vi "2_AdvancedDemo_HHHisto.vi"() -> ()   [LabVIEW 2020]
uses:
  Types/HH_InputChannel.ctl
  Types/HH_UIThread_Cmds.ctl
  Types/HH_UIThread_Data.ctl
  _lib/PQ/HydraHarp/HH_InitInfo.ctl
  _lib/PQ/HydraHarp/HH_RefSource.ctl
  _lib/PQ/HydraHarp/HH_MeasMode.ctl
  <vilib>/Utility/error.llb/DialogType.ctl
  _lib/PQ/HydraHarp/hhlib_x86_x64_UIThread.llb/HH_DllPath_global.vi
  <vilib>/Utility/error.llb/Error Cluster From Error Code.vi
  _lib/PQ/HydraHarp/HH_LibVersion_global.vi
  <vilib>/ErrorRing/Error Ring.xnode
panel:
  in  "Settings":bool=TRUE
  in  "Run continuously":bool=TRUE caption="Conti."
  in  "Start":bool
  in  "Scale":bool
  out "CountRates":i32[](graph)
  in  "HistoLength":i32(ring)=6 caption="Num Bins" items=["1024", "2048", "4096", "8192", "16384", "32768", "65536"]
  in  "OvlLevel":u32=4294967295 caption="Ovl.Level" min=1 step=1
  in  "StopOvl.":bool=TRUE
  in  "AcqTime":i32=1000 caption="Acqu.     ms" min=1 max=360000000 step=1
  in  "Binning":i32(ring) caption="Resol.      ps" items=["1", "2", "4", "8", "16", "32", "64", "128", "256", "512", "1024", "2048", "4096", "8192", "16384", "32768", "65536", "131072", "262144", "524288", "1048576", "2097152", "4194304", "8388608", "16777216", "33554432"]
  in  "HistoOffset":i32 caption="Offset      ns" min=0 max=500000 step=1
  out "HistoGraph":T1(graph)={0.0, "Resolution"=0.001, "Histogram"=array8x1024[8192 elements]}
  in  "SyncZeroX":i32=10 caption="ZeroCr.  mV" min=0 max=40 step=1
  in  "SyncDivider":i32(ring)=3 caption="Divider" items=["1", "2", "4", "8", "16"]
  in  "SyncOffset":i32 caption="Offset      ps" min=-99999 max=99999 step=1
  in  "SyncLevel":i32=50 caption="Level      mV" min=0 max=1000 step=1
  in  "Channels":T2[](array[typedef])=[{"Name"="Inp.Chan 1", "Enable"=TRUE, "Offset"=0, "CFDLevel"=50, "ZeroX"=10}, {"Name"="Inp.Chan 2", "Enable"=TRUE, "Offset"=0, "CFDLevel"=50, "ZeroX"=10}, {"Name"="Inp.Chan 3", "Enable"=TRUE, "Offset"=0, "CFDLevel"=50, "ZeroX"=10}, {"Name"="Inp.Chan 4", "Enable"=TRUE, "Offset"=0, "CFDLevel"=50, "ZeroX"=10}, {"Name"="Inp.Chan 5", "Enable"=TRUE, "Offset"=0, "CFDLevel"=50, "ZeroX"=10}, {"Name"="Inp.Chan 6", "Enable"=TRUE, "Offset"=0, "CFDLevel"=50, "ZeroX"=10}, {"Name"="Inp.Chan 7", "Enable"=TRUE, "Offset"=0, "CFDLevel"=50, "ZeroX"=10}, {"Name"="Inp.Chan 8", "Enable"=TRUE, "Offset"=0, "CFDLevel"=50, "ZeroX"=10}] {"ZeroX" min=0 max=40 step=1; "Offset" min=-99999 max=99999 step=1; "CFDLevel" min=0 max=1000 step=1}
  out "SyncRate":string="Sync Rate: 0 cps\n"
  out "OverFlow":bool caption="Overflow:"
  out "Status":string="Initialized!"
  # "Histogram"
  # "Sync"
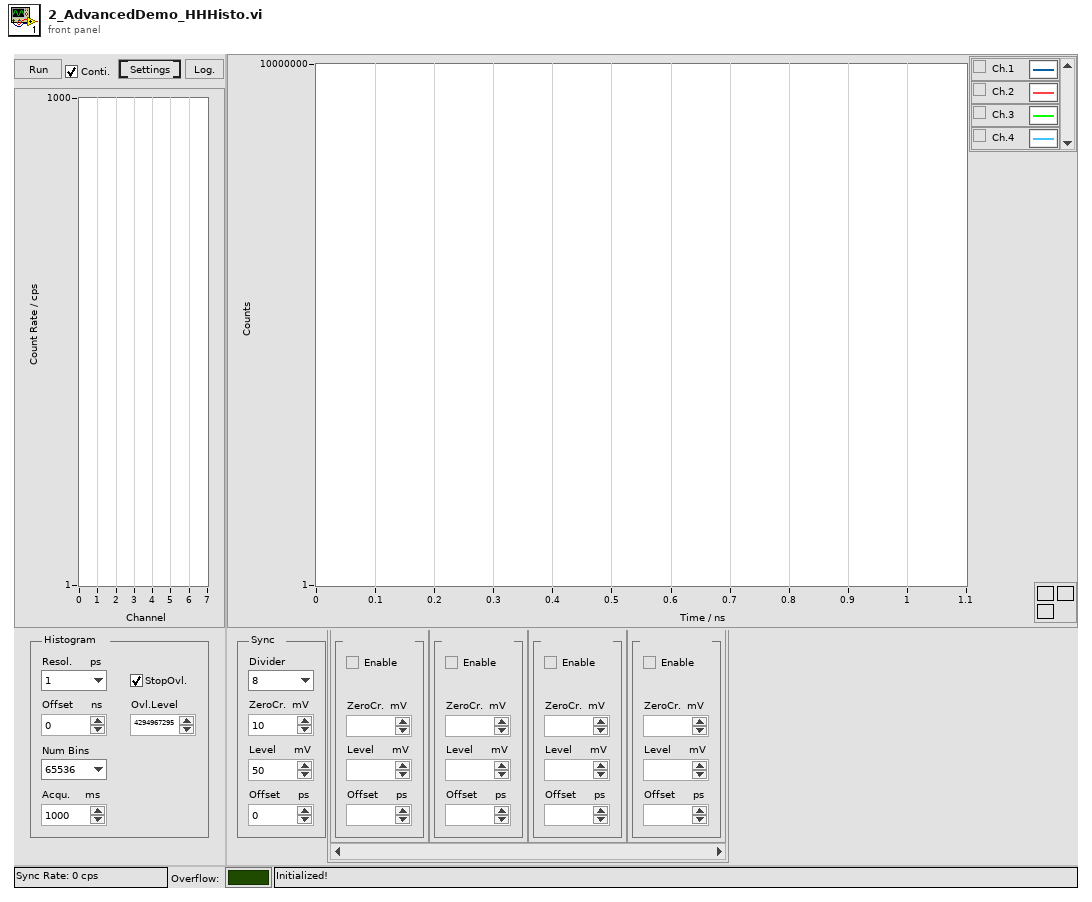
[diagram p1: front panel]
types:
  T1 = cluster{dbl, "Resolution":dbl, "Histogram":u32[][]}
  T2 = typedef "HH_InputChannel.ctl" = cluster{"Name":string, "Enable":bool, "Offset":i32, "CFDLevel":i32, "ZeroX":i32}
  T3 = typedef "HH_UIThread_Data.ctl" = cluster{"Init Info":T4, "DevIdx":i32, "SyncDivider":i32, "SyncOffset":i32, "SyncLevel":i32, "Channels":T2[], "CurrentChannels":i32[], "AcqTime":i32, "Binning":i32, "HistoOffset":i32, "HistoLen":i32, "StopOvl.":bool, "OvlLevel":u32, "StartMeas":bool, "HistoLength":i32, "Resolution":dbl, "Run cont.":bool, "Status":string, "SyncRate":i32, "BitShift":i32, "HistoAcqTime":dbl, "SyncZeroX":i32, "SyncRateStart":i32}
  T4 = typedef "HH_InitInfo.ctl" = cluster{"Library Version":string, "Serial No.":string, "Model":string, "Partnum":string, "Version":string, "features":i32, "nchannels":i32, "nummod":i32, "Model Codes":i32[], "Version Codes":i32[], "Base Resolution":dbl, "Bin Steps":i32}
  T5 = typedef "HH_UIThread_Cmds.ctl" = enum16{"Idle", "Init", "SetInpChanEnable", "SetInpChanOffset", "SetInpChanTrg", "SetSyncDivider", "SetSyncTrg", "SetSyncOffset", "SetBinning", "SetHistoOffset", "SetHistoLen", "SetStopOvl", "SetBitShift", "SetHistoAcqTime", "GetRates", "StartMeas", "StopMeas", "AbortMeas", "GetResolution", "GetHisto", "ReadFiFo", "WriteStatus", "Resize", "EnableControls", "DisableControls", "Error", "Exit"}
  T6 = enum8{"Enabled", "Disabled", "Disabled and Grayed Out"}
  T7 = typedef "HH_MeasMode.ctl" = i32
  T8 = typedef "HH_RefSource.ctl" = enum16{"internal", "external"}
  T9 = typedef "DialogType.ctl" = u16
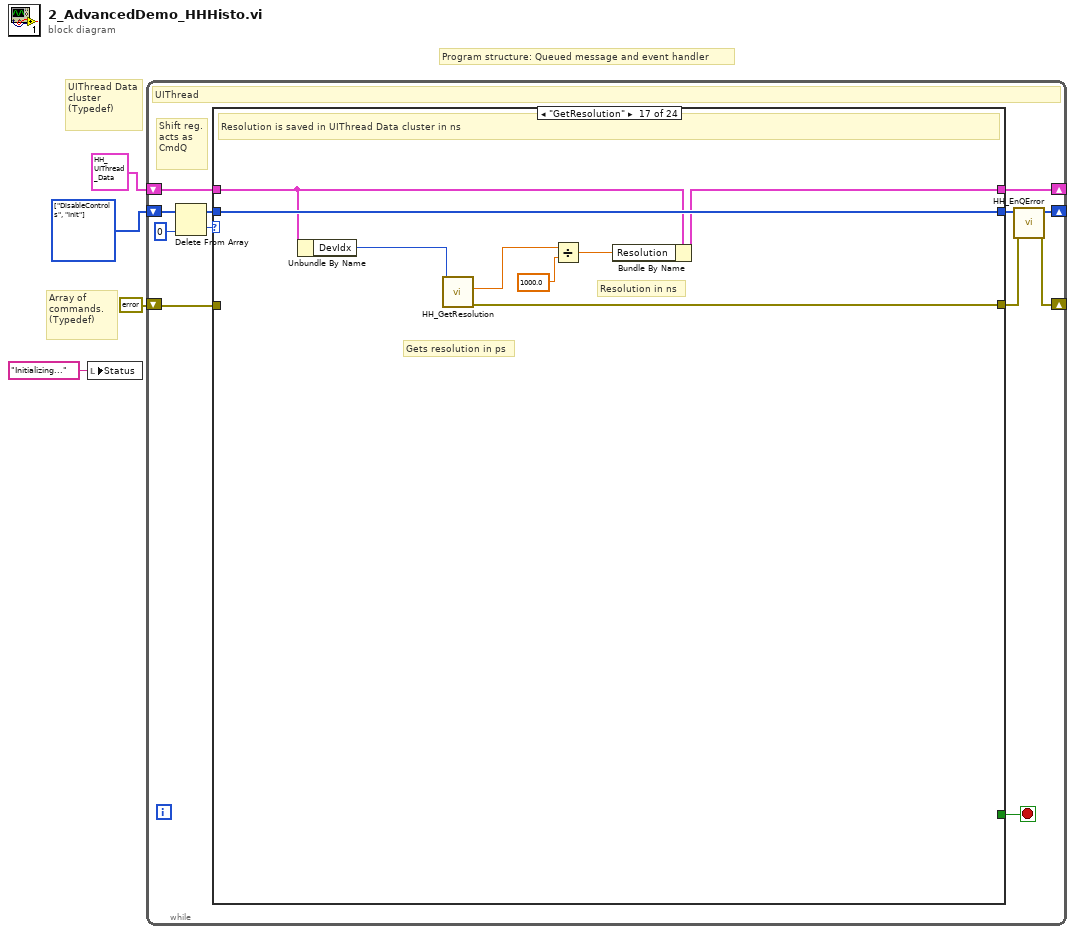
[diagram p0: block diagram]
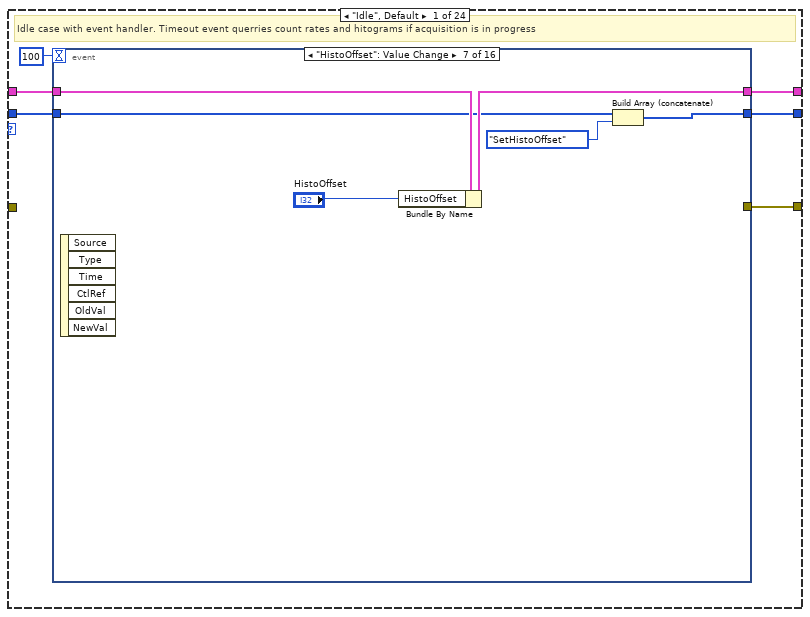
[diagram p2: hidden frame]
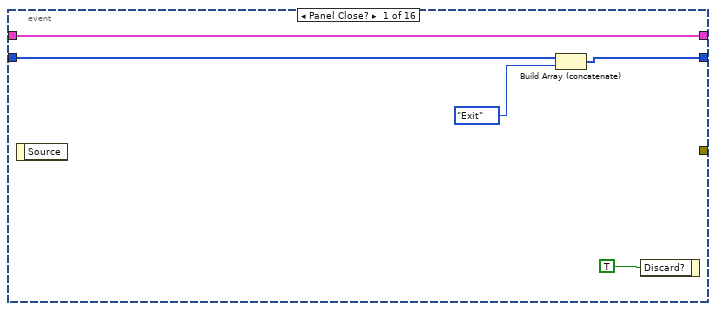
[diagram p3: hidden frame]
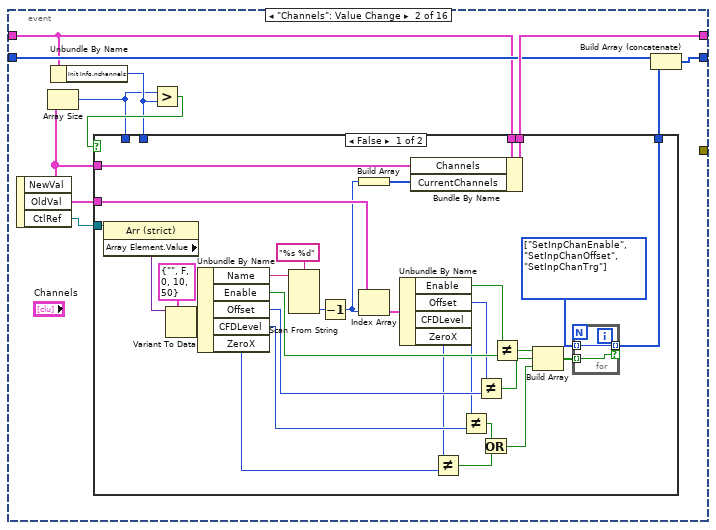
[diagram p4: hidden frame]
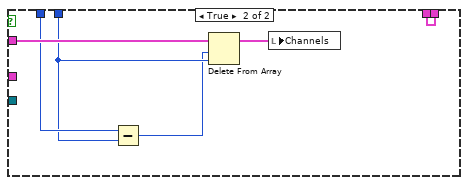
[diagram p5: hidden frame]
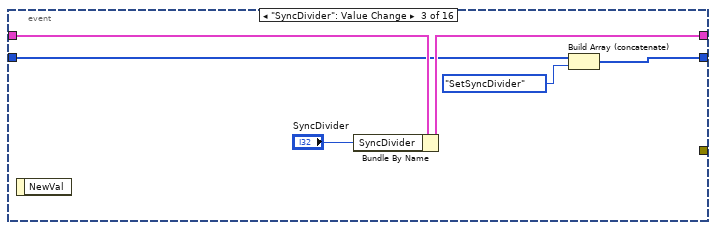
[diagram p6: hidden frame]
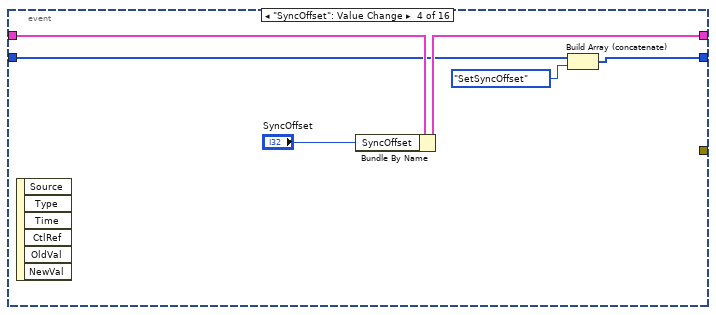
[diagram p7: hidden frame]
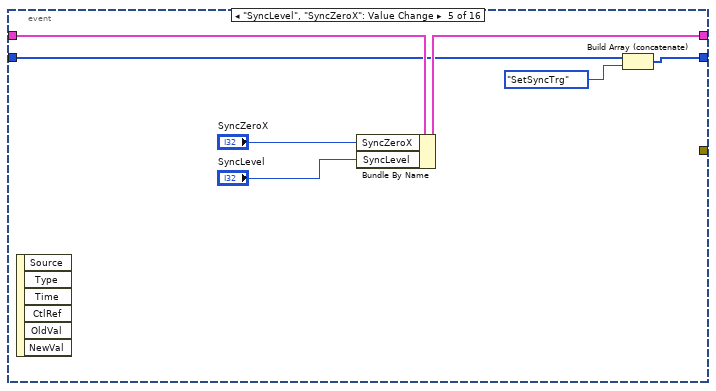
[diagram p8: hidden frame]
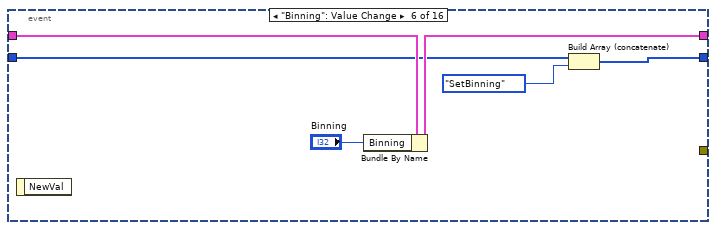
[diagram p9: hidden frame]
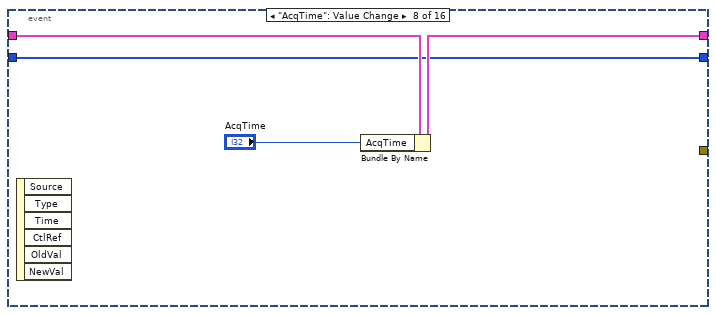
[diagram p10: hidden frame]
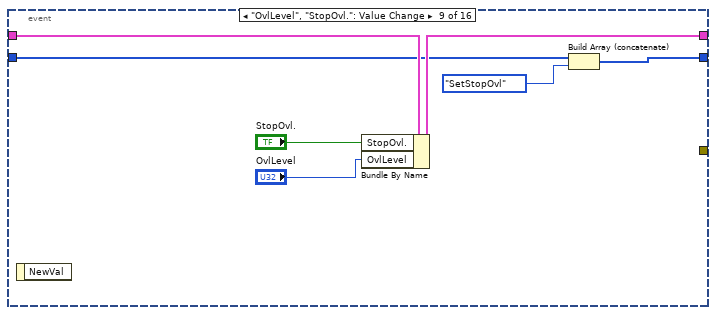
[diagram p11: hidden frame]
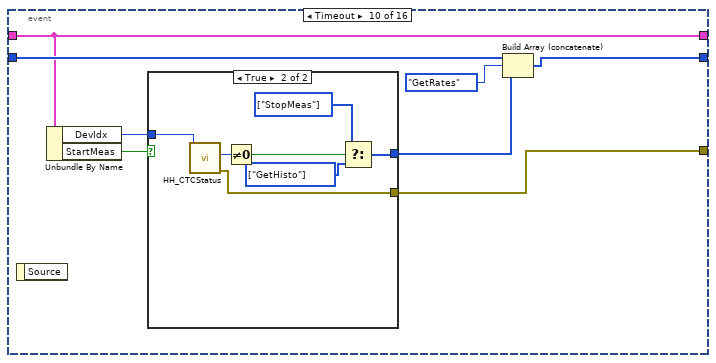
[diagram p12: hidden frame]
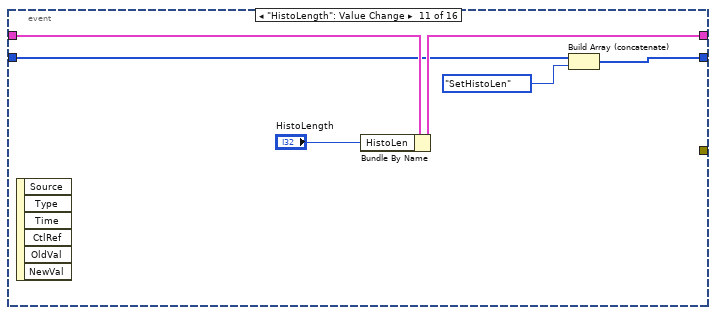
[diagram p14: hidden frame]
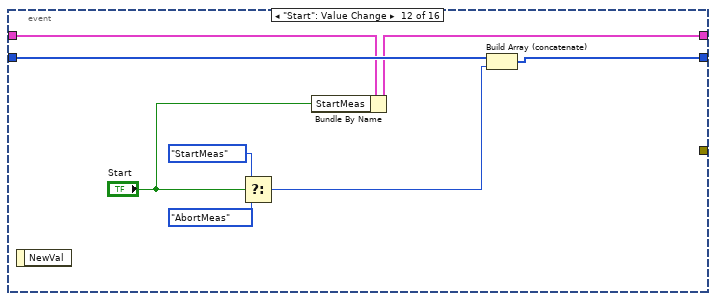
[diagram p15: hidden frame]
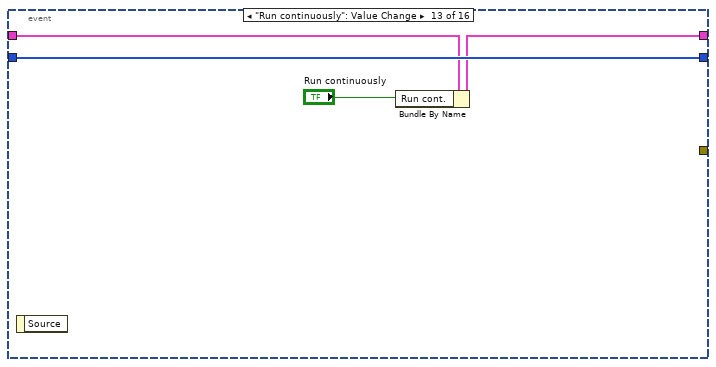
[diagram p16: hidden frame]
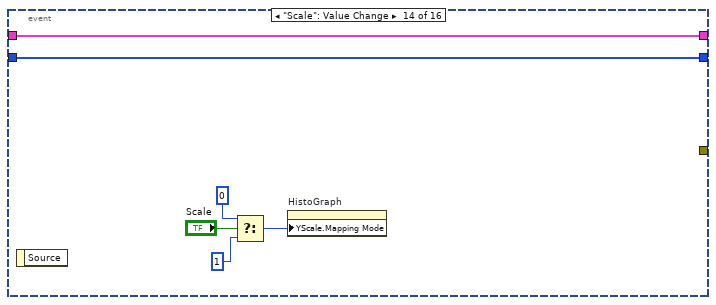
[diagram p17: hidden frame]
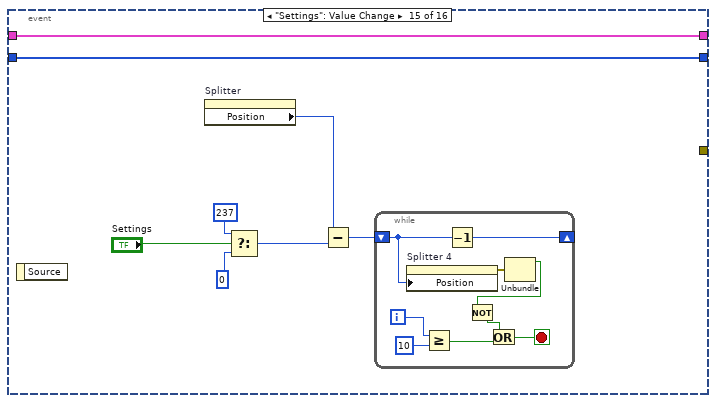
[diagram p18: hidden frame]
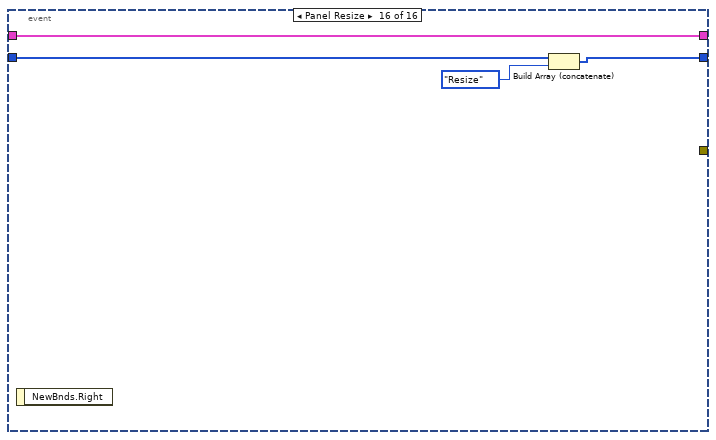
[diagram p19: hidden frame]
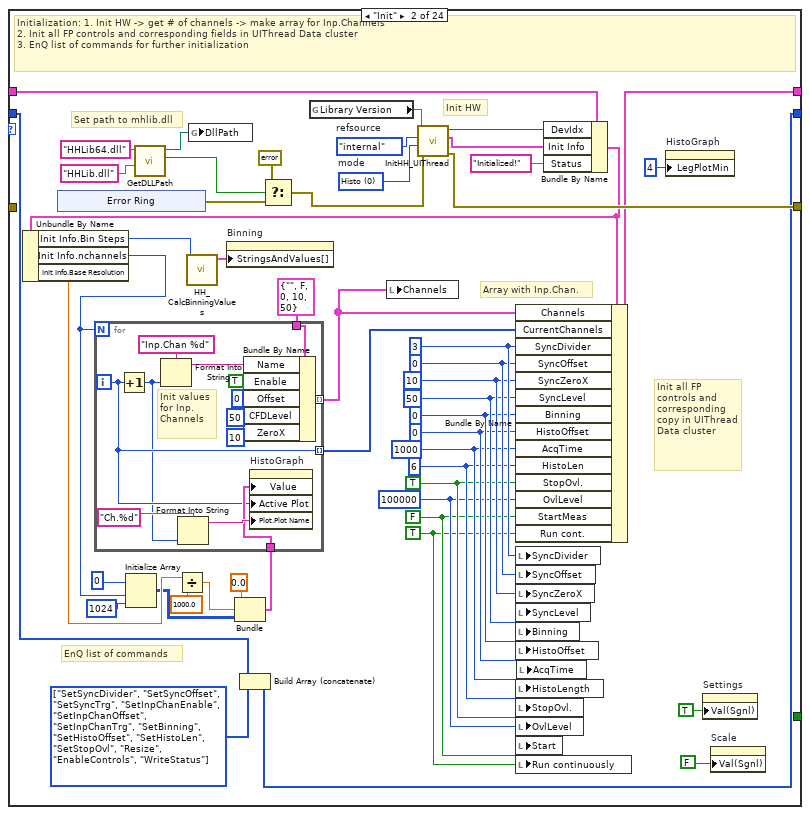
[diagram p20: hidden frame]
diagram:
  w3 = T5[] [enum."DisableControls", enum."Init"] items=["Idle", "Init", "SetInpChanEnable", "SetInpChanOffset", "SetInpChanTrg", "SetSyncDivider", "SetSyncTrg", "SetSyncOffset", "SetBinning", "SetHistoOffset", "SetHistoLen", "SetStopOvl", "SetBitShift", "SetHistoAcqTime", "GetRates", "StartMeas", "StopMeas", "AbortMeas", "GetResolution", "GetHisto", "ReadFiFo", "WriteStatus", "Resize", "EnableControls", "DisableControls", "Error", "Exit"]
  # "Array of commands.\n(Typedef)"
  # "Program structure: Queued message and event handler"
  # "UIThread Data cluster\n(Typedef)"
  n1 = local write "Status"("Initializing..." ("Status")) -> ()
  n2 = while {
    shift-right: [w5] -> _
    shift-left: w3 -> [w12]
    shift-right: [w15] -> _
    shift-left: T3 {"Init Info"={"Library Version"="", "Serial No."="", "Model"="", "Partnum"="", "Version"="", "features"=0, "nchannels"=0, "nummod"=0, "Model Codes"=[], "Version Codes"=[], "Base Resolution"=0.0, "Bin Steps"=0}, "DevIdx"=0, "SyncDivider"=1, "SyncOffset"=0, "SyncLevel"=50, "Channels"=[], "CurrentChannels"=[], "AcqTime"=1, "Binning"=1, "HistoOffset"=1, "HistoLen"=1024, "StopOvl."=FALSE, "OvlLevel"=1024, "StartMeas"=FALSE, "HistoLength"=0, "Resolution"=0.0, "Run cont."=FALSE, "Status"="", "SyncRate"=0, "BitShift"=0, "HistoAcqTime"=0.0, "SyncZeroX"=10, "SyncRateStart"=0} -> [w14]
    shift-right: [w7] -> _
    shift-left: errorcluster {"status"=FALSE, "code"=0, "source"=""} ("error IO") -> [w13]
    stop <- w16 stop-if-true
    # "Shift reg.\nacts as\nCmdQ"
    # "UIThread"
    n3 = Delete From Array(array=w12, index=0) -> (deleted portion=w10:T5, array with subset deleted=w9:T5[])  [unwired: 1 in]
    n4 = case shown="\"GetResolution\"" w10 {
      tunnel: [w22 w221 w249 w263 w277 w294 w303 w305 w312 w320 w328 w333 w345 w360 w368 w382 w396 w421 w446 w459 w466 w478 w484 w488] -> w6
      tunnel: [_ _ _ _ _ _ _ _ _ _ _ _ _ _ _ _ _ _ _ _ _ _ _ TRUE] -> w16
      tunnel: [w21 w201 w252 w266 w280 w296 w304 w309 w316 w321 w323 w334 w344 w366 w371 w385 w392 w420 w445 w447 w465 w477 w485 w491] -> w15
      tunnel: w14 -> [w20 w206 w252 w266 w280 w296 w304 w309 w316 w321 w324 w334 w344 w366 w372 w386 w393 w420 w445 w447 w465 w477 w485 w491]
      tunnel: [w17 w224 w250 w264 w278 w292 w302 w308 w315 w319 w327 w332 w343 w365 w374 w388 w394 w416 _ _ _ _ _ w489] -> w8
      tunnel: w13 -> [_ _ _ _ _ _ _ _ _ _ _ _ _ _ _ _ _ _ _ _ _ _ w486 _]
      tunnel: w9 -> [w19 w223 w249 w263 w277 w294 w303 w305 w311 w320 w328 w333 w345 w361 w369 w383 w396 w421 w446 w459 w466 w478 _ w488]
      frame "Idle", Default {
        # "Idle case with event handler. Timeout event querries count rates and hitograms if acquisition is in progress"
        n5 = event shown="[6] \"HistoOffset\": Value Change" {
          selector: _ -> [_ _ _ _ _ _ _ _ _ _ _ _ _ _ _ _]
          dyn-events: _ -> [_ _ _ _ _ _ _ _ _ _ _ _ _ _ _ _]
          timeout: 100 -> [_ _ _ _ _ _ _ _ _ _ _ _ _ _ _ _]
          tunnel: [w23 w33 w77 w83 w90 w97 w103 w108 w114 w124 w135 w143 w151 w157 w165 w175] -> w22
          tunnel: [w26 w36 w81 w87 w94 w100 w106 w110 w117 w123 w138 w141 w149 w156 w164 w178] -> w21
          tunnel: w20 -> [w26 w32 w82 w88 w95 w101 w107 w111 w118 w123 w139 w142 w150 w156 w164 w178]
          tunnel: w19 -> [w25 w35 w79 w85 w92 w99 w105 w108 w116 w126 w137 w145 w151 w157 w165 w176]
          tunnel: [_ _ _ _ _ _ _ _ _ w119 _ _ _ _ _ _] -> w17
          event Panel Close? {
            n6 = event-data() -> ()  [unwired: 1 in, 1 out]
            n7 = Build Array (concatenate)(w25, HH_UIThread_Cmds."Exit") -> (w23:T5[])
            n8 = event-data("Discard?"=TRUE) -> ()  [unwired: 1 in, 1 out]
          }
          event "Channels": Value Change {
            n9 = event-data() -> ("NewVal"=w31:T2[], "OldVal"=w37:T2[], "CtlRef"=w38:refnum<vi>)  [unwired: 1 in]
            n10 = Array Size(array=w31) -> (size(s)=w28:i32)
            n11 = Unbundle By Name(w32) -> ("Init Info.nchannels"=w29:i32)
            n12 = Greater?(x=w28, y=w29) -> (0:w30:bool)
            n13 = case shown="False" w30 {
              tunnel: w38 -> [w68 _]
              tunnel: w37 -> [w62 _]
              tunnel: [w45 w76] -> w36
              tunnel: [w43 _] -> w34
              tunnel: w32 -> [w40 w76]
              tunnel: w31 -> [w39 w75]
              tunnel: w29 -> [_ w73]
              tunnel: w28 -> [_ w74]
              frame False {
                w46 = T5[] [enum."SetInpChanEnable", enum."SetInpChanOffset", enum."SetInpChanTrg"] items=["Idle", "Init", "SetInpChanEnable", "SetInpChanOffset", "SetInpChanTrg", "SetSyncDivider", "SetSyncTrg", "SetSyncOffset", "SetBinning", "SetHistoOffset", "SetHistoLen", "SetStopOvl", "SetBitShift", "SetHistoAcqTime", "GetRates", "StartMeas", "StopMeas", "AbortMeas", "GetResolution", "GetHisto", "ReadFiFo", "WriteStatus", "Resize", "EnableControls", "DisableControls", "Error", "Exit"]
                n14 = property class="Arr (strict)"(reference=w68) -> ("Array Element.Value"=w67:variant)  [unwired: 1 in, 2 out]
                n15 = Variant To Data(type=T2 {"Name"="", "Enable"=FALSE, "Offset"=0, "CFDLevel"=10, "ZeroX"=50} ("Channel"), Variant=w67) -> (data=w44:T2)  [unwired: 1 in, 1 out]
                n16 = Unbundle By Name(w44) -> ("Name"=w65:string, "Enable"=w59:bool, "Offset"=w57:i32, "CFDLevel"=w55:i32, "ZeroX"=w53:i32)
                n17 = Scan From String(format string="%s %d", input string=w65) -> (output 2=w63:i32)  [unwired: 5 in, 3 out]
                n18 = Decrement(x=w63) -> (x-1=w42:i32)
                n19 = Build Array(w42) -> (w41:i32[])
                n20 = Index Array(array=w62, index=w42) -> (element=w61:T2)
                n21 = Unbundle By Name(w61) -> ("Enable"=w60:bool, "Offset"=w58:i32, "CFDLevel"=w56:i32, "ZeroX"=w54:i32)
                n22 = Bundle By Name(cluster=w40, "Channels"=w39, "CurrentChannels"=w41) -> (w45:T3)
                n23 = Not Equal?(x=w54, y=w53) -> (x != y?=w48:bool)
                n24 = Not Equal?(x=w56, y=w55) -> (x != y?=w49:bool)
                n25 = Not Equal?(x=w58, y=w57) -> (x != y?=w51:bool)
                n26 = Or(x=w49, y=w48) -> (x .or. y?=w47:bool)
                n27 = Not Equal?(x=w60, y=w59) -> (x != y?=w52:bool)
                n28 = Build Array(w52, w51, w47) -> (w50:bool[])
                n29 = for {
                  tunnel: w50 -> [w69] mode=indexing
                  tunnel: w46 -> [w70] mode=indexing
                  tunnel: [w70] -> w43 mode=indexing if=w69
                }
              }
              frame True {
                n30 = Subtract(x=w74, y=w73) -> (x-y=w72:i32)
                n31 = Delete From Array(array=w75, length=w72, index=w73) -> (array with subset deleted=w71:T2[])  [unwired: 1 out]
                n32 = local write "Channels"(w71) -> ()
              }
            }
            n33 = Build Array (concatenate)(w35, w34) -> (w33:T5[])
          }
          event "SyncDivider": Value Change {
            n34 = event-data() -> ()  [unwired: 1 in, 1 out]
            n35 = Bundle By Name(cluster=w82, "SyncDivider"="SyncDivider") -> (w81:T3)
            n36 = Build Array (concatenate)(w79, HH_UIThread_Cmds."SetSyncDivider") -> (w77:T5[])
          }
          event "SyncOffset": Value Change {
            n37 = event-data() -> ()  [unwired: 1 in, 6 out]
            n38 = Bundle By Name(cluster=w88, "SyncOffset"="SyncOffset") -> (w87:T3)
            n39 = Build Array (concatenate)(w85, HH_UIThread_Cmds."SetSyncOffset") -> (w83:T5[])
          }
          event "SyncLevel", "SyncZeroX": Value Change {
            n40 = event-data() -> ()  [unwired: 1 in, 6 out]
            n41 = Bundle By Name(cluster=w95, "SyncZeroX"="SyncZeroX", "SyncLevel"="SyncLevel") -> (w94:T3)
            n42 = Build Array (concatenate)(w92, HH_UIThread_Cmds."SetSyncTrg") -> (w90:T5[])
          }
          event "Binning": Value Change {
            n43 = event-data() -> ()  [unwired: 1 in, 1 out]
            n44 = Bundle By Name(cluster=w101, "Binning"="Binning") -> (w100:T3)
            n45 = Build Array (concatenate)(w99, HH_UIThread_Cmds."SetBinning") -> (w97:T5[])
          }
          event "HistoOffset": Value Change {
            n46 = event-data() -> ()  [unwired: 1 in, 6 out]
            n47 = Bundle By Name(cluster=w107, "HistoOffset"="HistoOffset") -> (w106:T3)
            n48 = Build Array (concatenate)(w105, HH_UIThread_Cmds."SetHistoOffset") -> (w103:T5[])
          }
          event "AcqTime": Value Change {
            n49 = event-data() -> ()  [unwired: 1 in, 6 out]
            n50 = Bundle By Name(cluster=w111, "AcqTime"="AcqTime") -> (w110:T3)
          }
          event "OvlLevel", "StopOvl.": Value Change {
            n51 = event-data() -> ()  [unwired: 1 in, 1 out]
            n52 = Bundle By Name(cluster=w118, "StopOvl."="StopOvl.", "OvlLevel"="OvlLevel") -> (w117:T3)
            n53 = Build Array (concatenate)(w116, HH_UIThread_Cmds."SetStopOvl") -> (w114:T5[])
          }
          event Timeout {
            n54 = event-data() -> ()  [unwired: 1 in, 1 out]
            n55 = Unbundle By Name(w123) -> ("DevIdx"=w121:i32, "StartMeas"=w122:bool)
            n56 = case shown="True" w122 {
              tunnel: w121 -> [_ w133]
              tunnel: [_ w131] -> w120
              tunnel: [_ w128] -> w119
              frame False {
              }
              frame True {
                w129 = T5[] [enum."GetHisto"] items=["Idle", "Init", "SetInpChanEnable", "SetInpChanOffset", "SetInpChanTrg", "SetSyncDivider", "SetSyncTrg", "SetSyncOffset", "SetBinning", "SetHistoOffset", "SetHistoLen", "SetStopOvl", "SetBitShift", "SetHistoAcqTime", "GetRates", "StartMeas", "StopMeas", "AbortMeas", "GetResolution", "GetHisto", "ReadFiFo", "WriteStatus", "Resize", "EnableControls", "DisableControls", "Error", "Exit"]
                w130 = T5[] [enum."StopMeas"] items=["Idle", "Init", "SetInpChanEnable", "SetInpChanOffset", "SetInpChanTrg", "SetSyncDivider", "SetSyncTrg", "SetSyncOffset", "SetBinning", "SetHistoOffset", "SetHistoLen", "SetStopOvl", "SetBitShift", "SetHistoAcqTime", "GetRates", "StartMeas", "StopMeas", "AbortMeas", "GetResolution", "GetHisto", "ReadFiFo", "WriteStatus", "Resize", "EnableControls", "DisableControls", "Error", "Exit"]
                n57 = call "HH_CTCStatus.vi"("devidx"=w133) -> ("error out"=w128:errorcluster, "ctcstatus"=w132:i32)  [unwired: 8 in, 1 out]
                n58 = Not Equal To 0?(x=w132) -> (x != 0?=w127:bool)
                n59 = Select(t=w130, s=w127, f=w129) -> (s? t:f=w131:T5[])
              }
            }
            n60 = Build Array (concatenate)(w126, HH_UIThread_Cmds."GetRates", w120) -> (w124:T5[])
          }
          event "HistoLength": Value Change {
            n61 = event-data() -> ()  [unwired: 1 in, 6 out]
            n62 = Bundle By Name(cluster=w139, "HistoLen"="HistoLength") -> (w138:T3)
            n63 = Build Array (concatenate)(w137, HH_UIThread_Cmds."SetHistoLen") -> (w135:T5[])
          }
          event "Start": Value Change {
            n64 = event-data() -> ()  [unwired: 1 in, 1 out]
            n65 = Select(t=HH_UIThread_Cmds."StartMeas", s="Start", f=HH_UIThread_Cmds."AbortMeas") -> (s? t:f=w144:T5)
            n66 = Bundle By Name(cluster=w142, "StartMeas"="Start") -> (w141:T3)
            n67 = Build Array (concatenate)(w145, w144) -> (w143:T5[])
          }
          event "Run continuously": Value Change {
            n68 = event-data() -> ()  [unwired: 1 in, 1 out]
            n69 = Bundle By Name(cluster=w150, "Run cont."="Run continuously") -> (w149:T3)
          }
          event "Scale": Value Change {
            n70 = event-data() -> ()  [unwired: 1 in, 1 out]
            n71 = Select(t=u8 0 ("Y Scale.Mapping Mode"), s="Scale", f=u8 1 ("Y Scale.Mapping Mode")) -> (s? t:f=w152:u8)
            n72 = property on="HistoGraph" class="WFGraph (strict)"("YScale.Mapping Mode"=w152) -> ()  [unwired: 2 in, 2 out]
          }
          event "Settings": Value Change {
            n73 = event-data() -> ()  [unwired: 1 in, 1 out]
            n74 = property on="Splitter" class="Splitter"() -> ("Position"=w163:i32)  [unwired: 2 in, 2 out]
            n75 = Select(t=237 ("PosT"), s="Settings", f=0 ("PosF")) -> (s? t:f=w160:i32)
            n76 = Subtract(x=w163, y=w160) -> (x-y=w159:i32)
            n77 = while {
              shift-right: [w174] -> _
              shift-left: w159 -> [w167]
              i -> [w173]
              stop <- w170 stop-if-true
              n78 = property on="Splitter 4" class="Splitter"("Position"=w167) -> (error out=w166:errorcluster)  [unwired: 2 in, 1 out]
              n79 = Greater Or Equal?(x=w173, y=10) -> (x >= y?=w171:bool)
              n80 = Decrement(x=w167) -> (x-1=w174:i32)
              n81 = Unbundle(w166) -> ("status"=w169:bool)  [unwired: 2 out]
              n82 = Not(x=w169) -> (.not. x?=w168:bool)
              n83 = Or(x=w168, y=w171) -> (x .or. y?=w170:bool)
            }
          }
          event Panel Resize {
            n84 = event-data() -> ()  [unwired: 1 in, 1 out]
            n85 = Build Array (concatenate)(w176, HH_UIThread_Cmds."Resize") -> (w175:T5[])
          }
        }
      }
      frame "Init" {
        w193 = T7 0 items=["Histo"=0, "T2"=2, "T3"=3, "Conti"=8]  # mode
        w192 = HH_RefSource."internal"  # refsource
        w208 = TRUE ("Run cont.")
        w210 = FALSE ("StartMeas")
        w211 = u32 100000 ("OvlLevel")
        w212 = TRUE ("StopOvl.")
        w213 = 6 ("HistoLen")
        w214 = 1000 ("AcqTime")
        w215 = 0 ("HistoOffset")
        w216 = 0 ("Binning")
        w217 = 50 ("SyncLevel")
        w218 = 10 ("SyncZeroX")
        w219 = 0 ("SyncOffset")
        w220 = 3 ("SyncDivider")
        w222 = T5[] [enum."SetSyncDivider", enum."SetSyncOffset", enum."SetSyncTrg", enum."SetInpChanEnable", enum."SetInpChanOffset", enum."SetInpChanTrg", enum."SetBinning", enum."SetHistoOffset", enum."SetHistoLen", enum."SetStopOvl", enum."Resize", enum."EnableControls", enum."WriteStatus"] items=["Idle", "Init", "SetInpChanEnable", "SetInpChanOffset", "SetInpChanTrg", "SetSyncDivider", "SetSyncTrg", "SetSyncOffset", "SetBinning", "SetHistoOffset", "SetHistoLen", "SetStopOvl", "SetBitShift", "SetHistoAcqTime", "GetRates", "StartMeas", "StopMeas", "AbortMeas", "GetResolution", "GetHisto", "ReadFiFo", "WriteStatus", "Resize", "EnableControls", "DisableControls", "Error", "Exit"]
        # "Init HW"
        # "Set path to mhlib.dll"
        # "Init all FP controls and corresponding copy in UIThread Data cluster"
        # "EnQ list of commands"
        # "Array with Inp.Chan."
        # "Initialization: 1. Init HW -> get # of channels -> make array for Inp.Channels\n2. Init all FP controls and corresponding fields in UIThread Data cluster\n3. EnQ list of commands for further initialization"
        n86 = xnode "Error Ring"() -> ("error out"=w194:errorcluster)
        n87 = call "GetDLLPath.vi"("DllName_32bit"="HHLib.dll" ("name or relative path"), "DllName_64bit"="HHLib64.dll" ("name or relative path")) -> ("file exists?"=w196:bool, "DLLPath"=w197:path)  [unwired: 8 in]
        n88 = global write "HH_DllPath_global.vi" "DllPath"(w197) -> ()
        n89 = Build Array (concatenate)(w223, w222) -> (w221:T5[])
        n90 = Select(t=errorcluster {"status"=FALSE, "code"=0, "source"=""} ("error IO"), s=w196, f=w194) -> (s? t:f=w202:errorcluster)
        n91 = global read "HH_LibVersion_global.vi" "Library Version"() -> (w191:string)
        n92 = call "InitHH_UIThread.vi"("error in (no error)"=w202, "mode"=w193, "refsource"=w192, "Library Version"=w191) -> ("error out"=w224:errorcluster, "Init Info"=w227:T4, "DevIdx"=w226:i32)  [unwired: 5 in]
        n93 = local write "SyncDivider"(w220) -> ()
        n94 = local write "SyncOffset"(w219) -> ()
        n95 = local write "SyncZeroX"(w218) -> ()
        n96 = local write "SyncLevel"(w217) -> ()
        n97 = local write "Binning"(w216) -> ()
        n98 = local write "HistoOffset"(w215) -> ()
        n99 = local write "HistoLength"(w213) -> ()
        n100 = local write "StopOvl."(w212) -> ()
        n101 = local write "OvlLevel"(w211) -> ()
        n102 = local write "Start"(w210) -> ()
        n103 = local write "Run continuously"(w208) -> ()
        n104 = local write "AcqTime"(w214) -> ()
        n105 = Bundle By Name(cluster=w206, "DevIdx"=w226, "Init Info"=w227, "Status"="Initialized!") -> (w205:T3)
        n106 = Unbundle By Name(w205) -> ("Init Info.Bin Steps"=w204:i32, "Init Info.nchannels"=w180:i32, "Init Info.Base Resolution"=w185:dbl)
        n107 = Initialize Array(u32 0, w180, 1024 ("dimension size")) -> (w184:u32[][])
        n108 = Divide(x=w185, y=1000.0) -> (x/y=w186:dbl)
        n109 = call "HH_CalcBinningValues.vi"("Bin Steps"=w204) -> ("BinningValues"=w209:cluster{"String":string, "Value":i32}[])  [unwired: 10 in]
        n110 = property on="Binning" class="Ring (strict)"("StringsAndValues[]"=w209) -> ()  [unwired: 2 in, 2 out]
        n111 = Bundle(0.0, w186, w184) -> (w183:cluster{dbl, dbl, u32[][]})  [unwired: 1 in]
        n112 = for {
          N: w180 -> [_]
          tunnel: T2 {"Name"="", "Enable"=FALSE, "Offset"=0, "CFDLevel"=10, "ZeroX"=50} ("Channel") -> [w245]
          tunnel: [w244] -> w179 mode=indexing
          tunnel: [w234] -> w181 mode=indexing
          tunnel: w183 -> [w235]
          i -> [w234]
          # "Init values for Inp. Channels"
          n113 = Increment(x=w234) -> (x+1=w233:i32)
          n114 = Format Into String(format string="Inp.Chan %d", w233) -> (resulting string=w242:string)  [unwired: 2 in, 1 out]
          n115 = Format Into String(format string="Ch.%d", w233) -> (resulting string=w236:string)  [unwired: 2 in, 1 out]
          n116 = Bundle By Name(cluster=w245, "Name"=w242, "Enable"=TRUE, "Offset"=0, "CFDLevel"=50 ("CFDZeroX"), "ZeroX"=10 ("CFDLevel")) -> (w244:T2)
          n117 = property on="HistoGraph" class="WFGraph (strict)"("Value"=w235, "Active Plot"=w234, "Plot.Plot Name"=w236) -> ()  [unwired: 2 in, 2 out]
        }
        n118 = local write "Channels"(w179) -> ()
        n119 = Bundle By Name(cluster=w205, "Channels"=w179, "CurrentChannels"=w181, "SyncDivider"=w220, "SyncOffset"=w219, "SyncZeroX"=w218, "SyncLevel"=w217, "Binning"=w216, "HistoOffset"=w215, "AcqTime"=w214, "HistoLen"=w213, "StopOvl."=w212, "OvlLevel"=w211, "StartMeas"=w210, "Run cont."=w208) -> (w201:T3)
        n120 = property on="HistoGraph" class="WFGraph (strict)"("LegPlotMin"=u32 4 ("Legend:Plot Minimum")) -> ()  [unwired: 2 in, 2 out]
        n121 = property on="Settings" class="Bool (strict)"("Val(Sgnl)"=TRUE ("Value (Signaling)")) -> ()  [unwired: 2 in, 2 out]
        n122 = property on="Scale" class="Bool (strict)"("Val(Sgnl)"=FALSE ("Value (Signaling)")) -> ()  [unwired: 2 in, 2 out]
      }
      frame "SetInpChanEnable" {
        n123 = Unbundle By Name(w252) -> ("DevIdx"=w251:i32, "Channels"=w246:T2[], "CurrentChannels"=w247:i32[])
        n124 = for {
          tunnel: w251 -> [w259]
          shift-right: [w258] -> w250
          shift-left: errorcluster {"status"=FALSE, "code"=0, "source"=""} ("error out") -> [w257]
          tunnel: w247 -> [w253] mode=indexing
          tunnel: w246 -> [w256]
          n125 = Index Array(array=w256, index=w253) -> (element=w255:T2)
          n126 = Unbundle By Name(w255) -> ("Enable"=w254:bool)
          n127 = call "HH_SetInputChannelEnable.vi"("error in (no error)"=w257, "enable"=w254, "channel"=w253, "devidx"=w259) -> ("error out"=w258:errorcluster)  [unwired: 6 in, 1 out]
        }
      }
      frame "SetInpChanOffset" {
        n128 = Unbundle By Name(w266) -> ("DevIdx"=w265:i32, "Channels"=w260:T2[], "CurrentChannels"=w261:i32[])
        n129 = for {
          tunnel: w265 -> [w271]
          shift-right: [w268] -> w264
          shift-left: errorcluster {"status"=FALSE, "code"=0, "source"=""} ("error out") -> [w269]
          tunnel: w261 -> [w270] mode=indexing
          tunnel: w260 -> [w273]
          n130 = Index Array(array=w273, index=w270) -> (element=w272:T2)
          n131 = Unbundle By Name(w272) -> ("Offset"=w267:i32)
          n132 = call "HH_SetInputChannelOffset.vi"("error in (no error)"=w269, "Offset"=w267, "channel"=w270, "devidx"=w271) -> ("error out"=w268:errorcluster)  [unwired: 6 in, 1 out]
        }
      }
      frame "SetInpChanTrg" {
        n133 = Unbundle By Name(w280) -> ("DevIdx"=w279:i32, "Channels"=w274:T2[], "CurrentChannels"=w275:i32[])
        n134 = for {
          tunnel: w279 -> [w283]
          shift-right: [w285] -> w278
          shift-left: errorcluster {"status"=FALSE, "code"=0, "source"=""} ("error out") -> [w286]
          tunnel: w275 -> [w284] mode=indexing
          tunnel: w274 -> [w288]
          n135 = Index Array(array=w288, index=w284) -> (element=w287:T2)
          n136 = Unbundle By Name(w287) -> ("CFDLevel"=w282:i32, "ZeroX"=w281:i32)
          n137 = call "HH_SetInputCFD.vi"("CFD Channel"=w284, "error in (no error)"=w286, "CFD ZeroCross"=w281, "CFD Level"=w282, "devidx"=w283) -> ("error out"=w285:errorcluster)  [unwired: 5 in, 1 out]
        }
      }
      frame "SetSyncDivider" {
        n138 = Unbundle By Name(w296) -> ("DevIdx"=w295:i32, "SyncDivider"=w291:i32)
        n139 = Power Of 2(x=w291) -> (2^x=w290:dbl)
        n140 = To Long Integer(number=w290) -> (32bit integer=w289:i32)
        n141 = call "HH_SetSyncDiv.vi"("SyncDivider"=w289, "devidx"=w295) -> ("error out"=w293:errorcluster)  [unwired: 8 in, 1 out]
        n142 = flat-sequence {
          tunnel: w293 -> [w297]
          tunnel: [w297] -> w292
          frame #0 {
            n143 = Wait (ms)(milliseconds to wait=u32 100) -> ()  [unwired: 1 out]
          }
        }
      }
      frame "SetSyncTrg" {
        n144 = Unbundle By Name(w304) -> ("DevIdx"=w301:i32, "SyncLevel"=w299:i32, "SyncZeroX"=w300:i32)
        n145 = call "HH_SetSyncCFD.vi"("CFD ZeroCross"=w300, "CFD Level"=w299, "devidx"=w301) -> ("error out"=w302:errorcluster)  [unwired: 7 in, 1 out]
      }
      frame "SetSyncOffset" {
        n146 = Unbundle By Name(w309) -> ("DevIdx"=w307:i32, "SyncOffset"=w306:i32)
        n147 = call "HH_SetSyncChannelOffset.vi"("Offset"=w306, "devidx"=w307) -> ("error out"=w308:errorcluster)  [unwired: 8 in, 1 out]
      }
      frame "SetBinning" {
        # "When binning is changed the new resolution is querried"
        n148 = Unbundle By Name(w316) -> ("DevIdx"=w314:i32, "Binning"=w313:i32)
        n149 = call "HH_SetBinning.vi"("Binning"=w313, "devidx"=w314) -> ("error out"=w315:errorcluster)  [unwired: 8 in, 1 out]
        n150 = Build Array (concatenate)(HH_UIThread_Cmds."GetResolution", w311) -> (w312:T5[])
      }
      frame "SetHistoOffset" {
        n151 = Unbundle By Name(w321) -> ("DevIdx"=w318:i32, "HistoOffset"=w317:i32)
        n152 = call "HH_SetOffset.vi"("Offset"=w317, "devidx"=w318) -> ("error out"=w319:errorcluster)  [unwired: 8 in, 1 out]
      }
      frame "SetHistoLen" {
        n153 = Unbundle By Name(w324) -> ("DevIdx"=w326:i32, "HistoLen"=w325:i32)
        n154 = call "HH_SetHistoLen.vi"("lencode"=w325, "devidx"=w326) -> ("error out"=w327:errorcluster, "actuallen"=w322:i32)  [unwired: 7 in, 1 out]
        n155 = Bundle By Name(cluster=w324, "HistoLength"=w322) -> (w323:T3)
      }
      frame "SetStopOvl" {
        n156 = Unbundle By Name(w334) -> ("DevIdx"=w331:i32, "StopOvl."=w330:bool, "OvlLevel"=w329:u32)
        n157 = call "HH_SetStopOverflow.vi"("stopcount"=w329, "StopOnOverflow"=w330, "devidx"=w331) -> ("error out"=w332:errorcluster)  [unwired: 7 in, 1 out]
      }
      frame "GetRates" {
        n158 = Unbundle By Name(w344) -> ("Init Info.nchannels"=w342:i32, "Channels"=w335:T2[], "DevIdx"=w336:i32)
        n159 = call "HH_GetSyncRate.vi"("devidx"=w336) -> ("error out"=w341:errorcluster, "syncrate"=w340:i32)  [unwired: 8 in, 1 out]
        n160 = Format Into String(format string="Sync Rate: %d cps\n", w340) -> (resulting string=→"SyncRate":string)  [unwired: 2 in, 1 out]
        n161 = for {
          N: w342 -> [_]
          tunnel: w336 -> [w351]
          tunnel: [w348] -> w338 mode=indexing
          shift-right: [w350] -> w343
          shift-left: w341 -> [w352]
          tunnel: w335 -> [w347] mode=indexing
          i -> [w349]
          n162 = Unbundle By Name(w347) -> ("Enable"=w346:bool)
          n163 = case shown="False" w346 {
            tunnel: w352 -> [w353 w358]
            tunnel: w351 -> [_ w357]
            tunnel: [w353 w356] -> w350
            tunnel: w349 -> [_ w355]
            tunnel: [_ w354] -> w348
            frame False {
            }
            frame True {
              n164 = call "HH_GetCountRate.vi"("error in (no error)"=w358, "Channel"=w355, "devidx"=w357) -> ("error out"=w356:errorcluster, "rate"=w354:i32)  [unwired: 6 in, 1 out]
            }
          }
        }
        "CountRates" <- w338
      }
      frame "StartMeas" {
        n165 = Unbundle By Name(w366) -> ("AcqTime"=w362:i32, "DevIdx"=w363:i32)
        n166 = call "HH_ClearHistMem.vi"("devidx"=w363) -> ("error out"=w364:errorcluster)  [unwired: 9 in, 1 out]
        n167 = call "HH_StartMeas.vi"("error in (no error)"=w364, "tacq"=w362, "devidx"=w363) -> ("error out"=w365:errorcluster)  [unwired: 7 in, 1 out]
        n168 = Build Array (concatenate)(w361, HH_UIThread_Cmds."GetHisto") -> (w360:T5[])
      }
      frame "StopMeas" {
        n169 = Unbundle By Name(w372) -> ("Run cont."=w367:bool, "DevIdx"=w373:i32)
        n170 = call "HH_StopMeas.vi"("devidx"=w373) -> ("error out"=w374:errorcluster)  [unwired: 9 in, 1 out]
        n171 = case shown="True" w367 {
          tunnel: w372 -> [w378 w380]
          tunnel: [w377 w380] -> w371
          tunnel: [w375 w379] -> w370
          frame False {
            w375 = T5[] [enum."GetHisto"] items=["Idle", "Init", "SetInpChanEnable", "SetInpChanOffset", "SetInpChanTrg", "SetSyncDivider", "SetSyncTrg", "SetSyncOffset", "SetBinning", "SetHistoOffset", "SetHistoLen", "SetStopOvl", "SetBitShift", "SetHistoAcqTime", "GetRates", "StartMeas", "StopMeas", "AbortMeas", "GetResolution", "GetHisto", "ReadFiFo", "WriteStatus", "Resize", "EnableControls", "DisableControls", "Error", "Exit"]
            w376 = FALSE ("StartMeas")
            n172 = Bundle By Name(cluster=w378, "StartMeas"=w376) -> (w377:T3)
            n173 = local write "Start"(w376) -> ()
          }
          frame True {
            w379 = T5[] [enum."GetHisto", enum."StartMeas"] items=["Idle", "Init", "SetInpChanEnable", "SetInpChanOffset", "SetInpChanTrg", "SetSyncDivider", "SetSyncTrg", "SetSyncOffset", "SetBinning", "SetHistoOffset", "SetHistoLen", "SetStopOvl", "SetBitShift", "SetHistoAcqTime", "GetRates", "StartMeas", "StopMeas", "AbortMeas", "GetResolution", "GetHisto", "ReadFiFo", "WriteStatus", "Resize", "EnableControls", "DisableControls", "Error", "Exit"]
          }
        }
        n174 = Build Array (concatenate)(w369, w370) -> (w368:T5[])
      }
      frame "AbortMeas" {
        w384 = T5[] [enum."GetHisto"] items=["Idle", "Init", "SetInpChanEnable", "SetInpChanOffset", "SetInpChanTrg", "SetSyncDivider", "SetSyncTrg", "SetSyncOffset", "SetBinning", "SetHistoOffset", "SetHistoLen", "SetStopOvl", "SetBitShift", "SetHistoAcqTime", "GetRates", "StartMeas", "StopMeas", "AbortMeas", "GetResolution", "GetHisto", "ReadFiFo", "WriteStatus", "Resize", "EnableControls", "DisableControls", "Error", "Exit"]
        w381 = FALSE ("StartMeas")
        n175 = Unbundle By Name(w386) -> ("DevIdx"=w387:i32)
        n176 = call "HH_StopMeas.vi"("devidx"=w387) -> ("error out"=w388:errorcluster)  [unwired: 9 in, 1 out]
        n177 = Bundle By Name(cluster=w386, "StartMeas"=w381) -> (w385:T3)
        n178 = local write "Start"(w381) -> ()
        n179 = Build Array (concatenate)(w383, w384) -> (w382:T5[])
      }
      frame "GetResolution" {
        # "Resolution in ns"
        # "Gets resolution in ps"
        # "Resolution is saved in UIThread Data cluster in ns"
        n180 = Unbundle By Name(w393) -> ("DevIdx"=w395:i32)
        n181 = call "HH_GetResolution.vi"("devidx"=w395) -> ("error out"=w394:errorcluster, "resolution"=w391:dbl)  [unwired: 8 in, 1 out]
        n182 = Divide(x=w391, y=1000.0) -> (x/y=w389:dbl)
        n183 = Bundle By Name(cluster=w393, "Resolution"=w389) -> (w392:T3)
      }
      frame "GetHisto" {
        w405 = 1  # FLAG_OVERFLOW
        # "Provides a buffer (U32-array of length 'HistoLength') for histograms."
        n184 = Unbundle By Name(w420) -> ("Resolution"=w417:dbl, "Init Info.nchannels"=w397:i32, "Channels"=w398:T2[], "DevIdx"=w419:i32, "HistoLength"=w418:i32)
        n185 = call "HH_AllocateHistoBuffer.vi"("HistoLength"=w418) -> ("Buffer"=w411:u32[])  [unwired: 10 in]
        n186 = for {
          N: w397 -> [_]
          tunnel: w419 -> [w434]
          tunnel: [w431] -> w408 mode=indexing
          tunnel: w411 -> [w432]
          shift-right: [w433] -> w407
          shift-left: errorcluster {"status"=FALSE, "code"=0, "source"=""} ("error IO") -> [w425]
          shift-right: [w426] -> w400
          shift-left: "Total Counts:\t\t" -> [w424]
          tunnel: w398 -> [w423] mode=indexing
          i -> [w430]
          n187 = Unbundle By Name(w423) -> ("Enable"=w422:bool)
          n188 = case shown="True" w422 {
            tunnel: w434 -> [_ w443]
            tunnel: [w435 w442] -> w433
            tunnel: w432 -> [w436 w440]
            tunnel: [w436 w439] -> w431
            tunnel: w430 -> [_ w438]
            tunnel: w425 -> [w435 w437]
            frame False {
            }
            frame True {
              n189 = call "HH_GetHistogram.vi"("Chcount"=w440, "error in (no error)"=w437, "clear"=0, "channel"=w438, "devidx"=w443) -> ("error out"=w442:errorcluster, "Histogram"=w439:u32[])  [unwired: 4 in, 1 out]
            }
          }
          n190 = Add Array Elements(numeric array=w431) -> (sum=w427:u32)
          n191 = Increment(x=w430) -> (x+1=w428:i32)
          n192 = Format Into String(format string="Ch.%2d: %d cnts.\t\t", initial string=w424, w428, w427) -> (resulting string=w426:string)  [unwired: 1 in, 1 out]
        }
        n193 = call "CalcRate.vi"("Refresh(ms)"=u32 500) -> ("Rate / Hz"=w415:dbl)  [unwired: 8 in, 2 out]
        n194 = Format Into String(format string="Readout Rate: %.1f Hz\\t\\t", w415) -> (resulting string=w413:string)  [unwired: 2 in, 1 out]
        n195 = Concatenate Strings(w413, w400) -> (w412:string)
        n196 = Bundle(0.0, "Resolution"=w417, "Histogram"=w408) -> (→"HistoGraph":T1)  [unwired: 1 in]
        n197 = local write "Status"(w412) -> ()
        n198 = call "HH_GetFlags.vi"("error in (no error)"=w407) -> ("error out"=w416:errorcluster, "flags"=w404:i32)  [unwired: 8 in, 1 out]
        n199 = And(x=w405, y=w404) -> (x .and. y?=w406:i32)
        n200 = Not Equal To 0?(x=w406) -> (x != 0?=→"OverFlow":bool)
      }
      frame "WriteStatus" {
        n201 = Unbundle By Name(w445) -> ("Status"=→"Status":string)
      }
      frame "Resize" {
        n202 = property on="Pane 3" class="Pane"() -> ("Width"=w452:u32)  [unwired: 2 in, 2 out]
        n203 = Subtract(x=w452, y=i16 100 ("b")) -> (x-y=w458:u32)
        n204 = Unbundle By Name(w447) -> ("Init Info.nchannels"=w455:i32)
        n205 = Quotient & Remainder(x=w458, y=i16 99 ("m")) -> (floor(x/y)=w457:u32)  [unwired: 1 out]
        n206 = In Range and Coerce(upper limit=w455, x=w457, lower limit=4) -> (coerced(x)=w456:u32)  [unwired: 1 out]
        n207 = Equal?(x=w455, y=w456) -> (x = y?=w454:bool)
        n208 = Not(x=w454) -> (.not. x?=w453:bool)
        n209 = property on="Channels" class="Arr (strict)"("HorizScroll"=w453, "Number of Columns"=w456, "Index Values"=u32[] [0]) -> ()  [unwired: 2 in, 2 out]
      }
      frame "EnableControls" {
        n210 = property class="VI"() -> ("Panel"=w463:refnum<vi>)  [unwired: 2 in, 2 out]
        n211 = property class="Pnl"(reference=w463) -> ("Controls[]"=w462:refnum<vi>[])  [unwired: 1 in, 2 out]
        n212 = property class="Pnl"(reference=w463) -> ("Decos[]"=w464:refnum<vi>[])  [unwired: 1 in, 2 out]
        n213 = for {
          tunnel: w464 -> [w468] mode=indexing
          tunnel: TRUE -> [w467]
          n214 = property class="Decor"(reference=w468, "Visible"=w467) -> ()  [unwired: 1 in, 2 out]
        }
        n215 = for {
          tunnel: w462 -> [w471] mode=indexing
          tunnel: T6."Enabled" ("Disabled") -> [w470]
          tunnel: [w469] -> _
          n216 = property class="Ctl"(reference=w471, "DisabledEnum"=w470) -> (error out=w469:errorcluster)  [unwired: 1 in, 1 out]
        }
      }
      frame "DisableControls" {
        n217 = property class="VI"() -> ("Panel"=w475:refnum<vi>)  [unwired: 2 in, 2 out]
        n218 = property class="Pnl"(reference=w475) -> ("Controls[]"=w474:refnum<vi>[])  [unwired: 1 in, 2 out]
        n219 = property class="Pnl"(reference=w475) -> ("Decos[]"=w476:refnum<vi>[])  [unwired: 1 in, 2 out]
        n220 = for {
          tunnel: w476 -> [w480] mode=indexing
          tunnel: FALSE -> [w479]
          n221 = property class="Decor"(reference=w480, "Visible"=w479) -> ()  [unwired: 1 in, 2 out]
        }
        n222 = for {
          tunnel: w474 -> [w483] mode=indexing
          tunnel: T6."Disabled and Grayed Out" ("Disabled") -> [w482]
          tunnel: [w481] -> _
          n223 = property class="Ctl"(reference=w483, "DisabledEnum"=w482) -> (error out=w481:errorcluster)  [unwired: 1 in, 1 out]
        }
      }
      frame "Error" {
        w484 = T5[] [enum."Exit"] items=["Idle", "Init", "SetInpChanEnable", "SetInpChanOffset", "SetInpChanTrg", "SetSyncDivider", "SetSyncTrg", "SetSyncOffset", "SetBinning", "SetHistoOffset", "SetHistoLen", "SetStopOvl", "SetBitShift", "SetHistoAcqTime", "GetRates", "StartMeas", "StopMeas", "AbortMeas", "GetResolution", "GetHisto", "ReadFiFo", "WriteStatus", "Resize", "EnableControls", "DisableControls", "Error", "Exit"]
        w487 = T9 1 items=["no dialog", "OK message", "continue or stop message", "OK message + warnings", "continue/stop + warnings"] ("type of dialog (OK msg:1)")
        # "Error case: If an error occures the user is informed and the programm terminates. Add your own code to handle error events (e.g. exception lists, etc.)"
        n224 = call <vilib>:"Simple Error Handler.vi"("type of dialog (OK msg:1)"=w487, "error in (no error)"=w486) -> ()  [unwired: 3 in, 5 out]
      }
      frame "Exit" {
        n225 = Unbundle By Name(w491) -> ("DevIdx"=w490:i32)
        n226 = call "HH_CloseDevice.vi"("devidx"=w490) -> ("error out"=w489:errorcluster)  [unwired: 9 in, 1 out]
      }
    }
    n227 = call "HH_EnQError.vi"("error in (no error)"=w8, "Cmds_in"=w6) -> ("error out"=w7:errorcluster, "Cmds_out"=w5:T5[])  [unwired: 8 in]
  }
